vi "Choreo_Choreo_SwerveCommand.vi"(4 "Pass_Through_Time":dbl=-1.0 format="%33.4f", 5 "TimePastEndSeconds":dbl=3.0, 6 "MirrorForRedAlliance":bool, 7 "ChoreoSwerveControlConfig":T7={"X_Adv PID Tuning"={"Kf"=0.0, "Kp"=3.0, "Ki"=0.0, "Kd"=0.0, "MaximumIntegral"=9.9e+30, "MinimumIntegral"=-9.9e+30, "Filter Derivative"=FALSE}, "X_Adv PID Limits"={"MaxInput"=0.0, "MinInput"=0.0, "Continuous"=FALSE, "MaxOutput"=9.9e+32, "MinOutput"=-9.9e+32}, "Y_Adv PID Tuning"={"Kf"=0.0, "Kp"=4.0, "Ki"=0.0, "Kd"=0.0, "MaximumIntegral"=9.9e+30, "MinimumIntegral"=-9.9e+30, "Filter Derivative"=FALSE}, "Y_Adv PID Limits"={"MaxInput"=0.0, "MinInput"=0.0, "Continuous"=FALSE, "MaxOutput"=9.9e+32, "MinOutput"=-9.9e+32}, "Rot_Adv PID Tuning"={"Kf"=0.0, "Kp"=5.0, "Ki"=0.0, "Kd"=0.0, "MaximumIntegral"=9.9e+30, "MinimumIntegral"=-9.9e+30, "Filter Derivative"=FALSE}, "Rot_Adv PID Limits"={"MaxInput"=3.141592653589793, "MinInput"=-3.14159, "Continuous"=TRUE, "MaxOutput"=9.9e+32, "MinOutput"=-9.9e+32}, "X Y Pos Tolerance M"=0.0381, "Rot Tolerance Deg"=0.0523599, "X Y Vel Tolerance M/S"=1.0, "Rot Vel Tolerance Deg/S"=30.0}, 8 "Auto":bool=TRUE, 9 "Initialize":bool, 10 "ChoreoTrajectory":T5, 11 "Current Position":T2={"TRANSLATION"={"X"=0.0, "Y"=0.0}, "ROTATION"={"VALUE"=0.0, "COS"=1.0, "SIN"=0.0}} {"ROTATION"."SIN" format="%13.4f"; "ROTATION"."COS" format="%13.4f"; "ROTATION"."VALUE" format="%13.4f"; "TRANSLATION"."Y" format="%14.3f"; "TRANSLATION"."X" format="%14.3f"}) -> (1 "Complete":bool, 2 "On Target":bool, 3 "Chassis Speed Dmd":T1 {"vOmega" format="%10.3f"; "vY" format="%10.3f"; "vX" format="%10.3f"})   [LabVIEW 2019, in "ChoreoLib.lvlib"]
uses:
  ChoreoLib.lvlib
  TypeDef/ChoreoSwerveControlConfig.ctl
  <vilib>/Rock Robotics/WPI/ThirdParty/JAS_Junk/TrajLib/TypeDef/PID_ADV_TUNING.ctl
  <vilib>/Rock Robotics/WPI/ThirdParty/JAS_Junk/TrajLib/TypeDef/PID_ADV_LIMITS.ctl
  TypeDef/ChoreoTrajectory.ctl
  TypeDef/ChoreoTrajectoryState.ctl
  <vilib>/Rock Robotics/WPI/ThirdParty/JAS_Junk/TrajLib/TypeDef/POSE2D.ctl
  <vilib>/Rock Robotics/WPI/ThirdParty/JAS_Junk/TrajLib/TypeDef/TRANSLATION2D.ctl
  <vilib>/Rock Robotics/WPI/ThirdParty/JAS_Junk/TrajLib/TypeDef/ROTATION2D.ctl
  <vilib>/Rock Robotics/WPI/ThirdParty/JAS_Junk/TrajLib/TypeDef/CHASSIS_SPEEDS.ctl
  <vilib>/Rock Robotics/WPI/DriverStation/WPI_DriverStationAllianceInfo.ctl
  <vilib>/Rock Robotics/WPI/ThirdParty/JAS_Junk/TrajLib/VI/Util_GetTime_U32.vi
  <vilib>/Rock Robotics/WPI/ThirdParty/JAS_Junk/TrajLib/VI/Util_GetTime_U64.vi
  <vilib>/Rock Robotics/WPI/ThirdParty/JAS_Junk/TrajLib/Trajectory_Library.lvlib
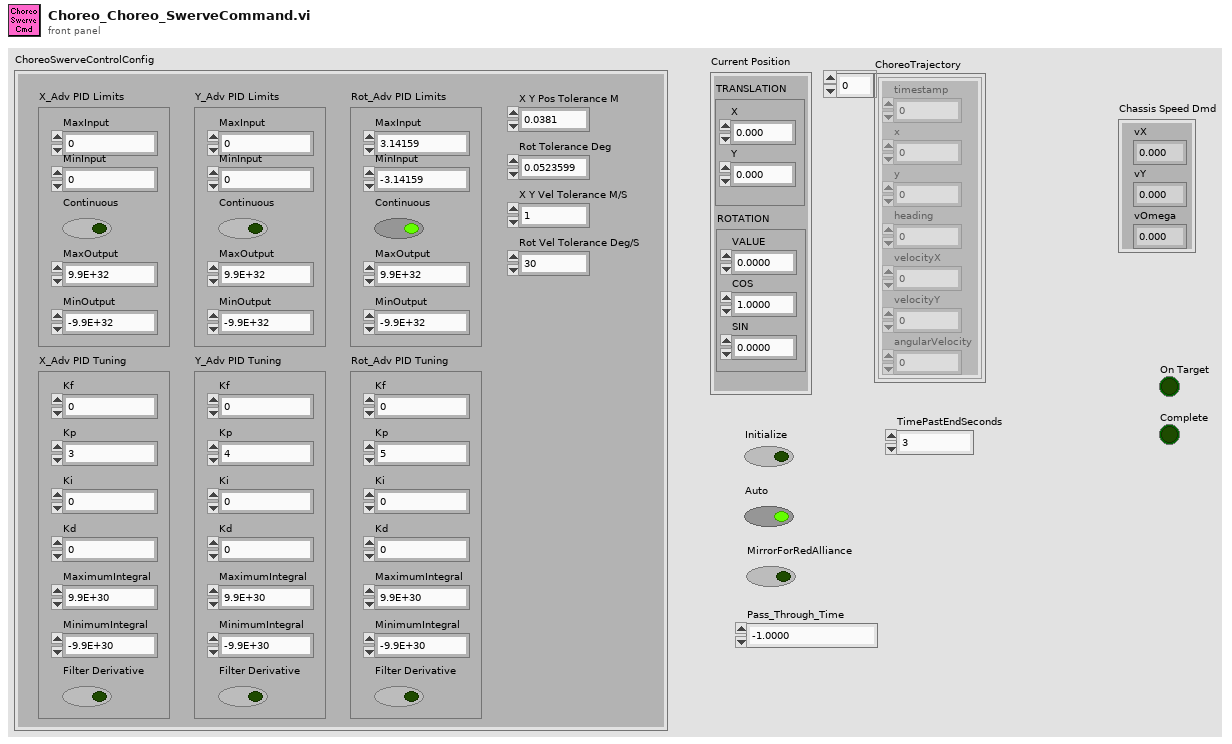
[diagram p1: front panel]
types:
  T1 = typedef "Trajectory_Library.lvlib/CHASSIS_SPEEDS.ctl" = cluster{"vX":dbl, "vY":dbl, "vOmega":dbl}
  T2 = typedef "Trajectory_Library.lvlib/POSE2D.ctl" = cluster{"TRANSLATION":T3, "ROTATION":T4}
  T3 = typedef "Trajectory_Library.lvlib/TRANSLATION2D.ctl" = cluster{"X":dbl, "Y":dbl}
  T4 = typedef "Trajectory_Library.lvlib/ROTATION2D.ctl" = cluster{"VALUE":dbl, "COS":dbl, "SIN":dbl}
  T5 = typedef "ChoreoLib.lvlib/ChoreoTrajectory.ctl" = T6[]
  T6 = typedef "ChoreoLib.lvlib/ChoreoTrajectoryState.ctl" = cluster{"timestamp":dbl, "x":dbl, "y":dbl, "heading":dbl, "velocityX":dbl, "velocityY":dbl, "angularVelocity":dbl}
  T7 = typedef "ChoreoLib.lvlib/ChoreoSwerveControlConfig.ctl" = cluster{"X_Adv PID Tuning":T8, "X_Adv PID Limits":T9, "Y_Adv PID Tuning":T8, "Y_Adv PID Limits":T9, "Rot_Adv PID Tuning":T8, "Rot_Adv PID Limits":T9, "X Y Pos Tolerance M":dbl, "Rot Tolerance Deg":dbl, "X Y Vel Tolerance M/S":dbl, "Rot Vel Tolerance Deg/S":dbl}
  T8 = typedef "Trajectory_Library.lvlib/PID_ADV_TUNING.ctl" = cluster{"Kf":dbl, "Kp":dbl, "Ki":dbl, "Kd":dbl, "MaximumIntegral":dbl, "MinimumIntegral":dbl, "Filter Derivative":bool}
  T9 = typedef "Trajectory_Library.lvlib/PID_ADV_LIMITS.ctl" = cluster{"MaxInput":dbl, "MinInput":dbl, "Continuous":bool, "MaxOutput":dbl, "MinOutput":dbl}
  T10 = typedef "WPI_DriverStationAllianceInfo.ctl" = enum16{"Red", "Blue", "Invalid"}
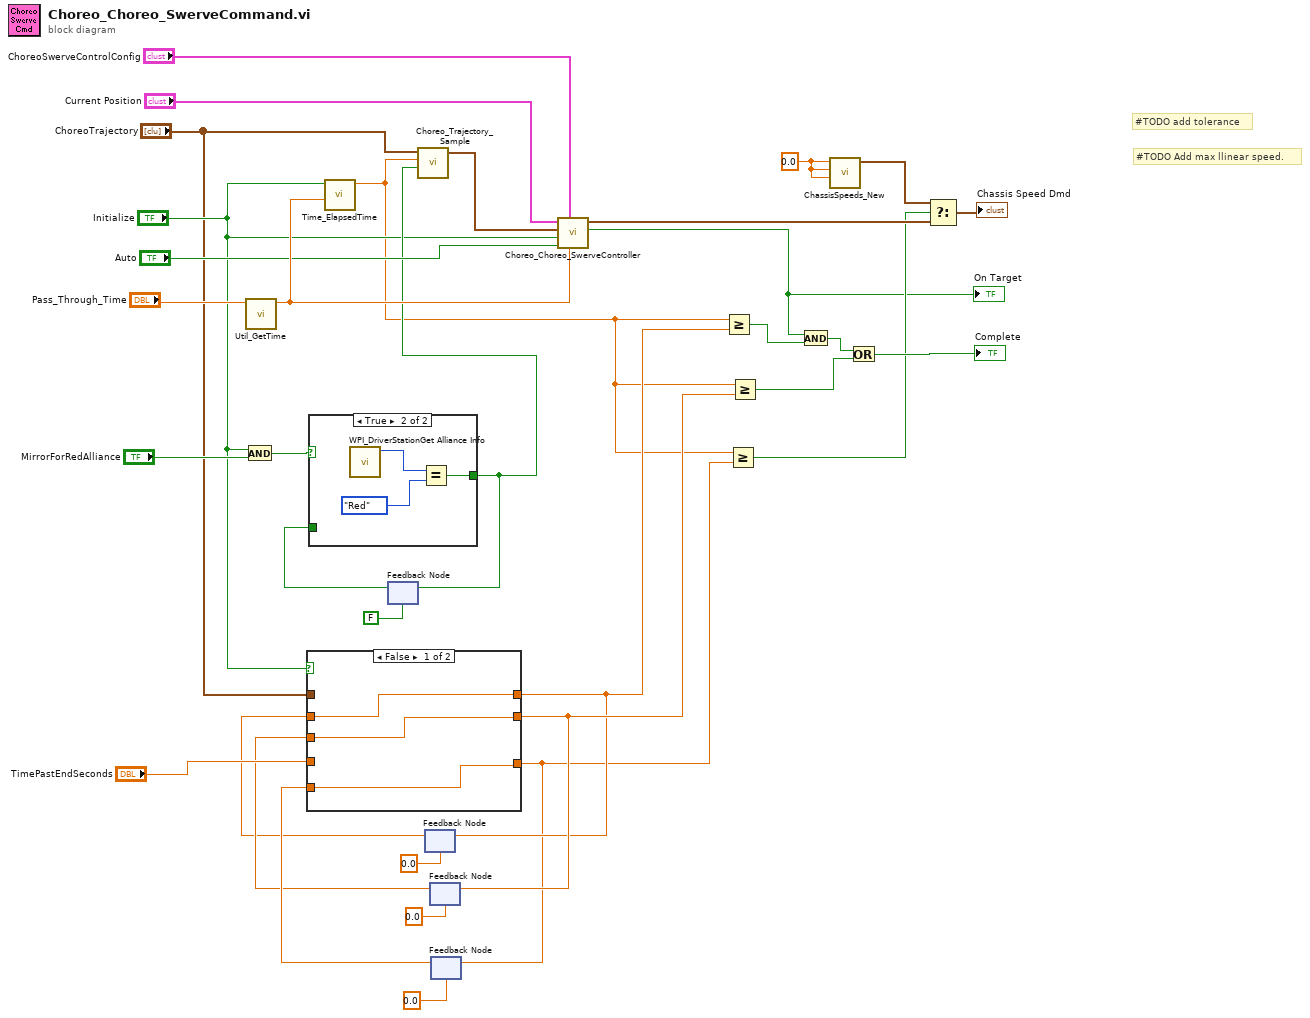
[diagram p0: block diagram]
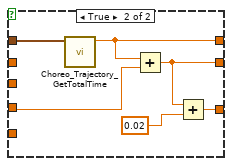
[diagram p2: hidden frame]
diagram:
  w3 = 0.0 ("vX")
  # "#TODO Add max llinear speed."
  # "#TODO add tolerance"
  n1 = And(x="Initialize", y="MirrorForRedAlliance") -> (x .and. y?=w27:bool)
  n2 = call <vilib>:"Util_GetTime.vi"("Pass_Through_Time"="Pass_Through_Time") -> ("FPGA_Time_Seconds"=w33:dbl)  [unwired: 8 in, 2 out]
  n3 = call <vilib>:"Time_ElapsedTime.vi"("PassthroughTime_SEC"=w33, "Reset"="Initialize") -> ("Elapsed Time Sec"=w9:dbl)  [unwired: 9 in]
  n4 = feedback #1(FALSE) -> (w25:bool)
  n5 = case shown="True" w27 {
    tunnel: [w35 w36] -> w24
    tunnel: w25 -> [w35 _]
    frame False {
    }
    frame True {
      n6 = call <vilib>:"WPI_DriverStationGet Alliance Info.vi"() -> ("Alliance"=w38:T10)  [unwired: 6 in, 5 out]
      n7 = Equal?(x=w38, y=WPI_DriverStationAllianceInfo."Red") -> (x = y?=w36:bool)
    }
  }
  n8 = feedback-in #1(w24) -> ()
  n9 = call "Choreo_Trajectory_Sample.vi"("MirrorForRedAlliance"=w24, "TimeStamp"=w9, "ChoreoTrajectory"="ChoreoTrajectory") -> ("ChoreoTrajectoryState"=w30:T6)  [unwired: 8 in]
  n10 = feedback #2(0.0) -> (w10:dbl)
  n11 = feedback #3(0.0) -> (w17:dbl)
  n12 = feedback #4(0.0) -> (w18:dbl)
  n13 = case shown="False" "Initialize" {
    tunnel: "ChoreoTrajectory" -> [_ w47]
    tunnel: "TimePastEndSeconds" -> [_ w46]
    tunnel: [w40 w45] -> w13
    tunnel: [w41 w43] -> w8
    tunnel: w18 -> [w41 _]
    tunnel: w17 -> [w40 _]
    tunnel: [w39 w42] -> w11
    tunnel: w10 -> [w39 _]
    frame False {
    }
    frame True {
      n14 = call "Choreo_Trajectory_GetTotalTime.vi"("ChoreoTrajectory"=w47) -> ("timestamp"=w42:dbl)  [unwired: 10 in]
      n15 = Add(x=w42, y=w46) -> (x+y=w45:dbl)
      n16 = Add(x=w45, y=0.02) -> (x+y=w43:dbl)
    }
  }
  n17 = feedback-in #2(w11) -> ()
  n18 = feedback-in #3(w13) -> ()
  n19 = feedback-in #4(w8) -> ()
  n20 = call "Choreo_Choreo_SwerveController.vi"("Pass_Through_Time"=w33, "ChoreoSwerveControlConfig"="ChoreoSwerveControlConfig", "Auto"="Auto", "Reset"="Initialize", "ChoreoTrajectoryState"=w30, "Current Position"="Current Position") -> ("On Target"=w1:bool, "Chassis Speed Dmd"=w7:T1)  [unwired: 4 in]
  "On Target" <- w1
  n21 = Greater Or Equal?(x=w9, y=w11) -> (x >= y?=w2:bool)
  n22 = Greater Or Equal?(x=w9, y=w8) -> (x >= y?=w6:bool)
  n23 = Greater Or Equal?(x=w9, y=w13) -> (x >= y?=w15:bool)
  n24 = And(x=w1, y=w2) -> (x .and. y?=w16:bool)
  n25 = call <vilib>:"ChassisSpeeds_New.vi"("vAngular"=w3, "vY"=w3, "vX"=w3) -> ("CHASSIS"=w4:T1)  [unwired: 8 in]
  n26 = Or(x=w16, y=w15) -> (x .or. y?=→"Complete":bool)
  n27 = Select(t=w4, s=w6, f=w7) -> (s? t:f=→"Chassis Speed Dmd":T1)
